vi "Segment_lateral_distance.vi"(9 "Turn Value (deg)":dbl, 10 "segment_trial_positions":dbl[](array[numeric]), 11 "Duration (cm)":string) -> (3 "Segment Lateral distance (total)":dbl)   [LabVIEW 2018]
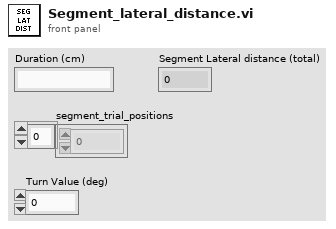
[diagram p1: front panel]
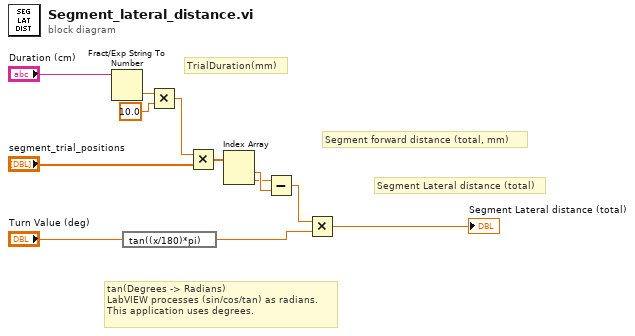
[diagram p0: block diagram]
diagram:
  # "Segment Lateral distance (total)"
  # "Segment forward distance (total, mm)"
  # "tan(Degrees -> Radians)\nLabVIEW processes (sin/cos/tan) as radians.\nThis application uses degrees."
  # "TrialDuration(mm)"
  n1 = Fract/Exp String To Number(string="Duration (cm)") -> (number=w8:dbl)  [unwired: 3 in, 1 out]
  n2 = expression code="tan((x/180)*pi)"("Turn Value (deg)") -> (w1:dbl)
  n3 = Multiply(x=w8, y=10.0) -> (x*y=w6:dbl)
  n4 = Multiply(x=w6, y="segment_trial_positions") -> (x*y=w4:dbl[])
  n5 = Index Array(array=w4) -> (element #1=w3:dbl, element #2=w2:dbl)  [unwired: 2 in]
  n6 = Subtract(x=w2, y=w3) -> (x-y=w5:dbl)
  n7 = Multiply(x=w5, y=w1) -> (x*y=→"Segment Lateral distance (total)":dbl)
